vi "Write Auth ID.vi"(8 "error in (no error)":errorcluster, 10 "Auth ID":string, 11 "SecretBasedAuthenticatorBase in":refnum<class "SecretBasedAuthenticatorBase.lvclass">) -> (0 "error out":errorcluster, 3 "SecretBasedAuthenticatorBase out":refnum<class "SecretBasedAuthenticatorBase.lvclass">)   [LabVIEW 2020, in "wamplv.lvlib" / "SecretBasedAuthenticatorBase.lvclass"]
uses:
  SecretBasedAuthenticatorBase.lvclass
  SecretBasedAuthenticatorBase.lvclass/SecretBasedAuthenticatorBase.ctl
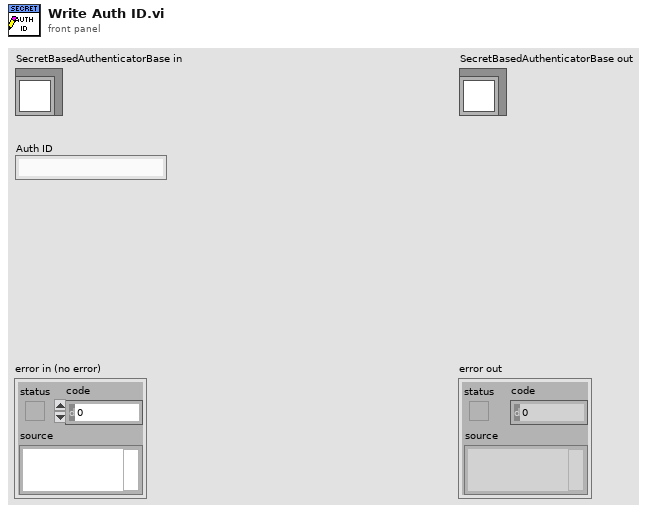
[diagram p1: front panel]
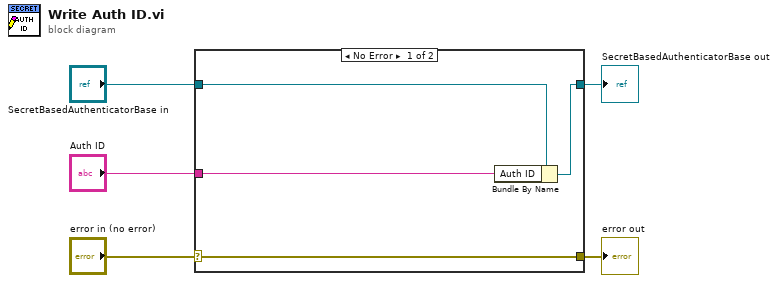
[diagram p0: block diagram]
diagram:
  n1 = case shown="No Error" "error in (no error)" {
    selector: "error in (no error)" -> [w9 w10]
    tunnel: [w9 w10] -> w4
    tunnel: [w7 w11] -> w2
    tunnel: "SecretBasedAuthenticatorBase in" -> [w8 w11]
    tunnel: "Auth ID" -> [w6 _]
    frame No Error {
      n2 = Bundle By Name(cluster=w8, "Auth ID"=w6) -> (w7:refnum<class "SecretBasedAuthenticatorBase.lvclass">)
    }
    frame Error {
    }
  }
  "error out" <- w4
  "SecretBasedAuthenticatorBase out" <- w2
